vi "GlobalEnableDisable.vi"(10 "DisableDeviceWebService":bool, 11 "action":enum16{"init", "set", "get"}(ring)=enum."get") -> (2 "DisableDeviceWebService":bool)   [LabVIEW 2017]
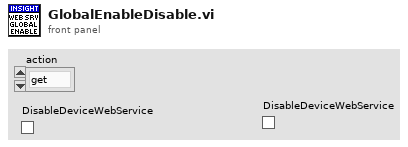
[diagram p1: front panel]
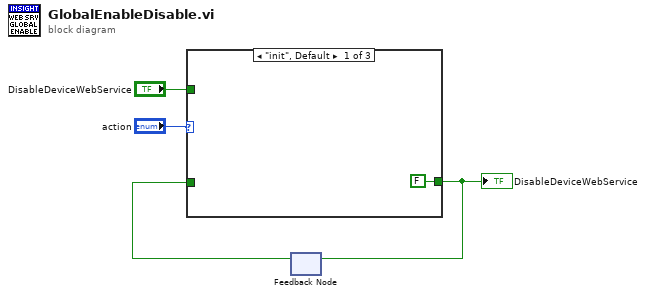
[diagram p0: block diagram]
diagram:
  n1 = feedback #1() -> (w1:bool)  [unwired: 1 in]
  n2 = case shown="\"init\", Default" "action" {
    tunnel: "DisableDeviceWebService" -> [_ w6 _]
    tunnel: [FALSE ("webservice enable in") w6 w7] -> w2
    tunnel: w1 -> [_ _ w7]
    frame "init", Default {
    }
    frame "set" {
    }
    frame "get" {
    }
  }
  "DisableDeviceWebService" <- w2
  n3 = feedback-in #1(w2) -> ()
